vi "1P結束.vi"(0 "結束":bool, 2 "青蛙數":dbl, 3 "您的分數":dbl) -> (1 "結束 2":bool)   [LabVIEW 2014]
panel:
  in  "再來一場":bool
  out "被您害死的青蛙 :":dbl
  out "您的分數 :":dbl
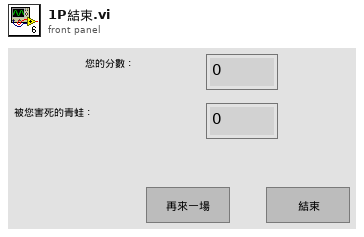
[diagram p1: front panel]
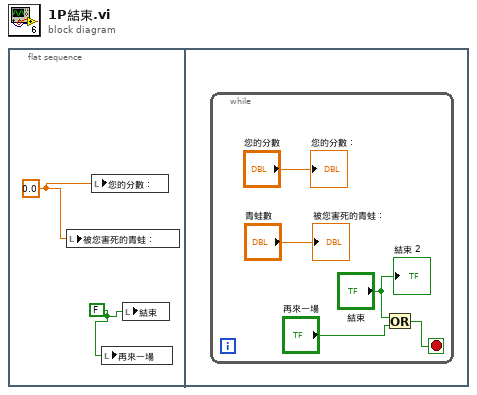
[diagram p0: block diagram]
diagram:
  n1 = flat-sequence {
    frame #0 {
      w1 = FALSE ("結束")
      w2 = 0.0
      n2 = local write "被您害死的青蛙 :"(w2) -> ()
      n3 = local write "您的分數 :"(w2) -> ()
      n4 = local write "再來一場"(w1) -> ()
      n5 = local write "結束"(w1) -> ()
    }
    frame #1 {
      n6 = while {
        stop <- w5 stop-if-true
        n7 = Or(x="結束", y="再來一場") -> (x .or. y?=w5:bool)
        "您的分數 :" <- "您的分數"
        "被您害死的青蛙 :" <- "青蛙數"
        "結束 2" <- "結束"
      }
    }
  }
